vi "Apply Parameters for FGen.vi"(6 "Acquire Rate":dbl, 7 "Sinewave Props":T1 {"Phase offset (deg)" format="%#_6p"; "Frequency (Hz)" format="%#_6p"}, 8 "error in (no error)":errorcluster, 9 "Wave Parameters":T1 {"Phase offset (deg)" format="%#_6p"; "Frequency (Hz)" format="%#_6p"}, 11 "Refnum in":refnum<k20>) -> (0 "error out":errorcluster, 1 "Actual loop rate 2":u32, 2 "Actual loop rate":u32, 3 "Refnum out":refnum<k20>)   [LabVIEW 2018]
uses:
  Program Files (x86)/National Instruments/LabVIEW 2018/ProjectTemplates/Source/myRIO/Oscilloscope/myRIO v1.1/Real-Time/Controls/Wave Parameters.ctl
  Program Files (x86)/National Instruments/LabVIEW 2018/ProjectTemplates/Source/myRIO/Oscilloscope/myRIO v1.1/Real-Time/Controls/Waveform Enum.ctl
  Program Files (x86)/National Instruments/LabVIEW 2018/ProjectTemplates/Source/myRIO/Oscilloscope/myRIO v1.1/Real-Time/Controls/Channel Selector.ctl
  <vilib>/rvi/Analysis/host/Private/Sample Rate To Loop Time (ticks).vi
  <vilib>/Utility/error.llb/Error Cluster From Error Code.vi
  <vilib>/rvi/errors/niLvFpgaAdjustHostInterfaceError.vi
  <vilib>/rvi/interface/nirviReadWriteControl/nirviReadWriteControl.xnode
  NiFpgaLv.dll
  <vilib>/rvi/interface/Simulation/niFpgaSimulationCallBeginRW.vi
  <vilib>/rvi/Analysis/host/Public/NI_FpgaMspHost.lvlib
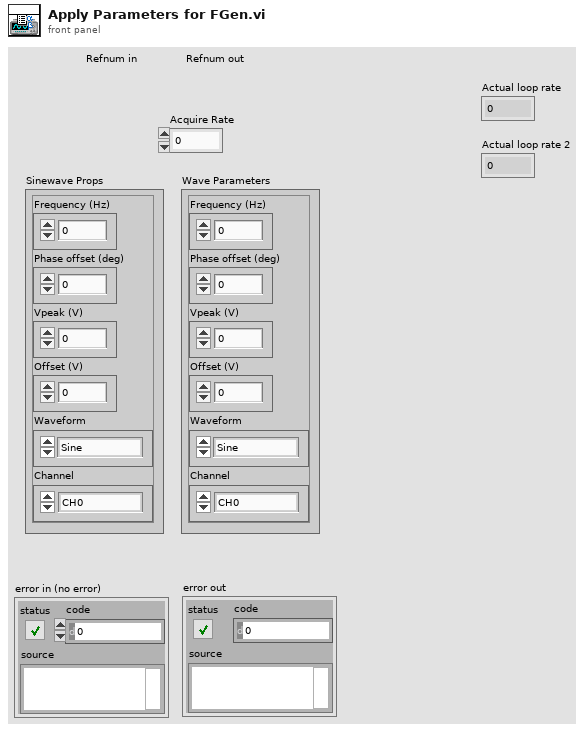
[diagram p1: front panel]
types:
  T1 = typedef "Wave Parameters.ctl" = cluster{"Frequency (Hz)":dbl, "Phase offset (deg)":dbl, "Vpeak (V)":dbl, "Offset (V)":dbl, "Waveform":T2, "Channel":T3}
  T2 = typedef "Waveform Enum.ctl" = enum16{"Sine", "Square"}
  T3 = typedef "Channel Selector.ctl" = enum16{"CH0", "CH1"}
  T4 = cluster{"Frequency (Hz)":bool, "Phase offset (deg)":bool, "Vpeak (V)":bool, "Offset (V)":bool, "Waveform":bool, "Channel":bool}
  T5 = typedef "Wave Properties - FPGA.ctl" = cluster{"Frequency (periods/tick)":fxp<+,32,0>, "Phase offset (periods)":fxp<+,32,0>, "Scale factor":fxp<+/-,24,1>, "Amplitude offset":fxp<+/-,24,12>, "Waveform":T2, "Channel":T3}
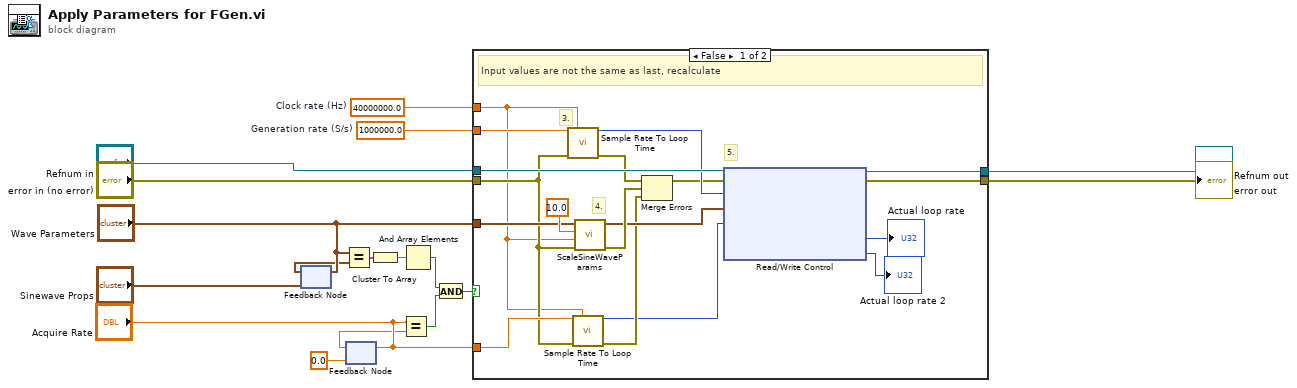
[diagram p0: block diagram]
diagram:
  w2 = 1000000.0  # Generation rate (S/s)
  w4 = 40000000.0  # Clock rate (Hz)
  n1 = feedback #1("Sinewave Props") -> (w8:T1)
  n2 = feedback-in #1("Wave Parameters") -> ()
  n3 = Equal?(x="Wave Parameters", y=w8) -> (x = y?=w6:T4)
  n4 = feedback #2(0.0 ("Acq Rate(us)")) -> (w11:dbl)
  n5 = feedback-in #2("Acquire Rate") -> ()
  n6 = Cluster To Array(cluster=w6) -> (array=w7:bool[])
  n7 = Equal?(x="Acquire Rate", y=w11) -> (x = y?=w13:bool)
  n8 = And Array Elements(Boolean array=w7) -> (logical AND=w14:bool)
  n9 = And(x=w14, y=w13) -> (x .and. y?=w15:bool)
  n10 = case shown="False" w15 {
    tunnel: "Refnum in" -> [w35 w37]
    tunnel: w2 -> [w33 _]
    tunnel: "error in (no error)" -> [w23 w36]
    tunnel: "Wave Parameters" -> [w25 _]
    tunnel: [w28 w37] -> w9
    tunnel: [w27 w36] -> w10
    tunnel: w4 -> [w20 _]
    tunnel: "Acquire Rate" -> [w24 _]
    frame False {
      # "3."
      # "5."
      # "4."
      # "Input values are not the same as last, recalculate"
      n11 = call-poly <vilib>:"Sample Rate To Loop Time.vi"("sample rate (S/s)"=w33, "FPGA clock rate (Hz)"=w20, "error in (no error)"=w23) -> ("count (ticks/S)"=w34:u32, "error out"=w30:errorcluster)  [unwired: 10 in, 1 out]
      n12 = call-poly <vilib>:"Sample Rate To Loop Time.vi"("sample rate (S/s)"=w24, "FPGA clock rate (Hz)"=w20, "error in (no error)"=w23) -> ("count (ticks/S)"=w21:u32, "error out"=w22:errorcluster)  [unwired: 10 in, 1 out]
      n13 = call "ScaleSineWaveParams.vi"("error in (no error)"=w23, "FPGA Clock Rate"=w20, "max voltage for target"=10.0, "Sine wave"=w25) -> ("error out"=w32:errorcluster, "Wave Props"=w26:T5)  [unwired: 6 in]
      n14 = Merge Errors(w30, w32, w22) -> (w31:errorcluster)
      n15 = xnode "Read/Write Control"("FPGA VI Reference In"=w35, "error in"=w31, "Desired loop rate (ticks)"=w34, "Wave Properties"=w26, "Acq Rate(ticks)"=w21) -> ("FPGA VI Reference Out"=w28:refnum<k20>, "error out"=w27:errorcluster, "Actual loop rate"=→"Actual loop rate":u32, "Actual loop rate 2"=→"Actual loop rate 2":u32)
    }
    frame True {
      # "Input values did not change, use previous values"
    }
  }
  "error out" <- w10
  "Refnum out" <- w9
